vi "cDAQ GET Module Temps.vi"(7 "NI Card Settings":T1, 8 "error in (no error)":errorcluster, 10 "Module Number":i32, 11 "Tasks (In)":refnum<k21>[](array[refnum])) -> (0 "error out":errorcluster, 1 "Raw Data":dbl[](array[numeric]) format="%0.2f", 2 "NI Module Data":string[][](array[string]), 3 "Tasks (Out)":refnum<k21>[](array[refnum]))   [LabVIEW 2019]
uses:
  Trunk/Washer DOE/Type Definitions/DOE Dryer NI Card Settings.ctl
  <vilib>/DAQmx/read.llb/DAQmx Read (Analog 1D DBL NChan 1Samp).vi
  <vilib>/DAQmx/miscellaneous.llb/DAQmx Fill In Error Info.vi
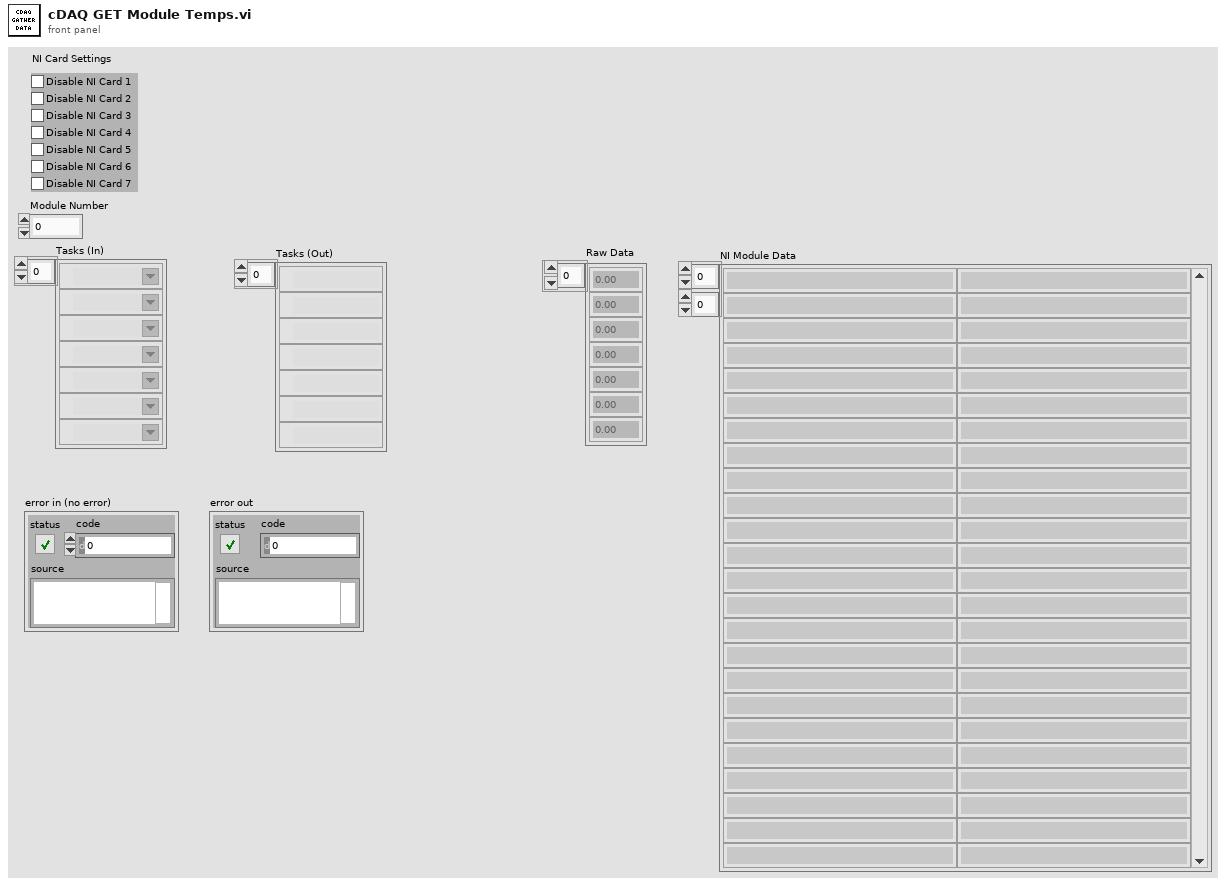
[diagram p1: front panel]
types:
  T1 = typedef "DOE Dryer NI Card Settings.ctl" = cluster{"Disable NI Card 1":bool, "Disable NI Card 2":bool, "Disable NI Card 3":bool, "Disable NI Card 4":bool, "Disable NI Card 5":bool, "Disable NI Card 6":bool, "Disable NI Card 7":bool}
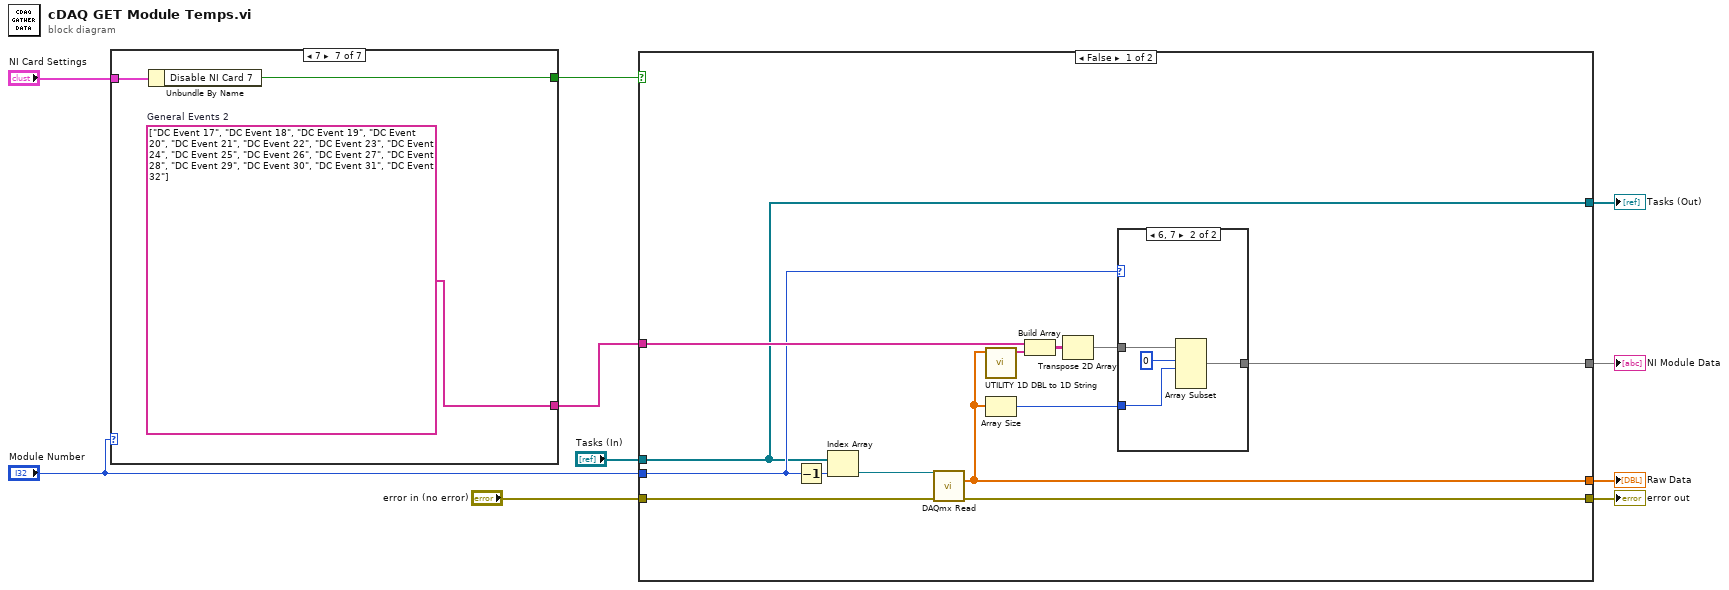
[diagram p0: block diagram]
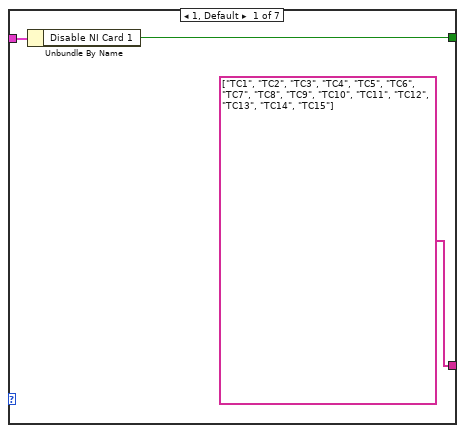
[diagram p2: hidden frame]
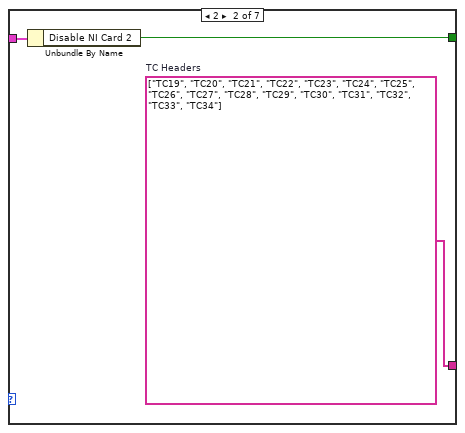
[diagram p3: hidden frame]
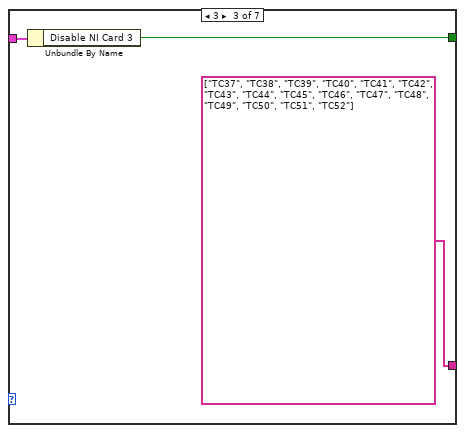
[diagram p4: hidden frame]
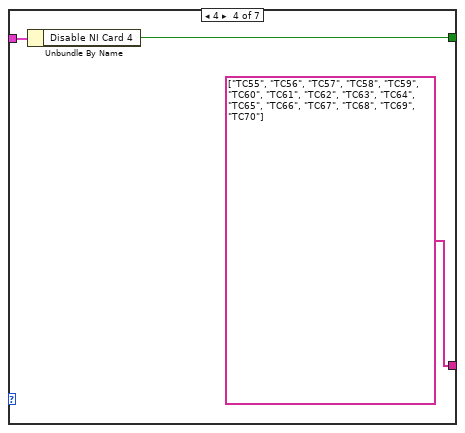
[diagram p5: hidden frame]
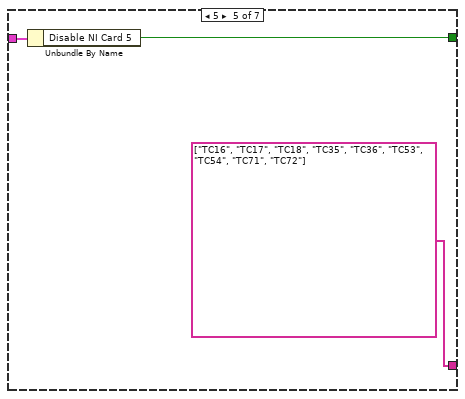
[diagram p6: hidden frame]
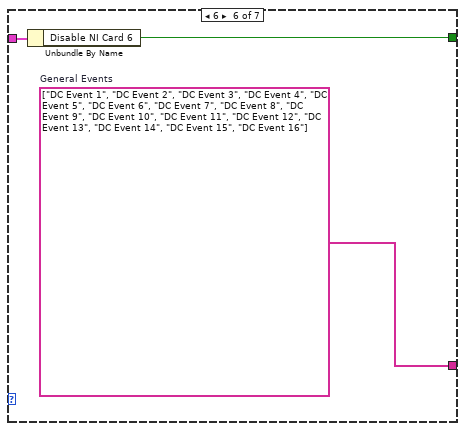
[diagram p7: hidden frame]
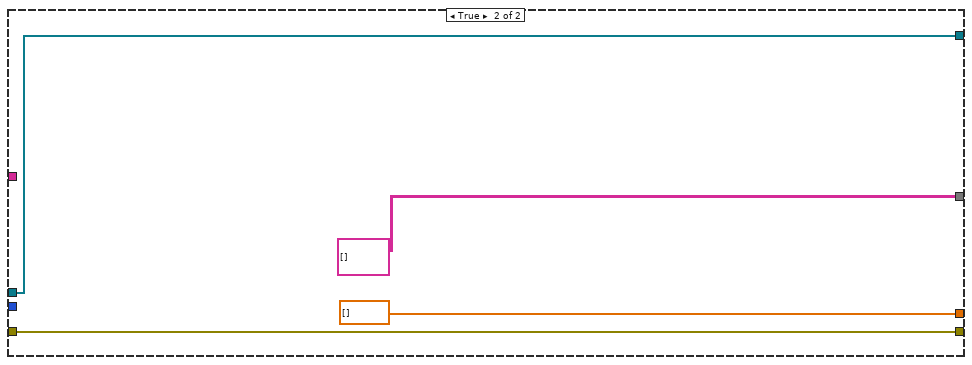
[diagram p9: hidden frame]
diagram:
  n1 = case shown="7" "Module Number" {
    tunnel: "NI Card Settings" -> [w13 w16 w19 w22 w25 w28 w31]
    tunnel: [w12 w15 w18 w21 w24 w27 w30] -> w4
    tunnel: [string[] ["TC1", "TC2", "TC3", "TC4", "TC5", "TC6", "TC7", "TC8", "TC9", "TC10", "TC11", "TC12", "TC13", "TC14", "TC15"] w14 string[] ["TC37", "TC38", "TC39", "TC40", "TC41", "TC42", "TC43", "TC44", "TC45", "TC46", "TC47", "TC48", "TC49", "TC50", "TC51", "TC52"] string[] ["TC55", "TC56", "TC57", "TC58", "TC59", "TC60", "TC61", "TC62", "TC63", "TC64", "TC65", "TC66", "TC67", "TC68", "TC69", "TC70"] string[] ["TC16", "TC17", "TC18", "TC35", "TC36", "TC53", "TC54", "TC71", "TC72"] w26 w29] -> w2
    frame 1, Default {
      n2 = Unbundle By Name(w13) -> ("Disable NI Card 1"=w12:bool)
    }
    frame 2 {
      w14 = string[] ["TC19", "TC20", "TC21", "TC22", "TC23", "TC24", "TC25", "TC26", "TC27", "TC28", "TC29", "TC30", "TC31", "TC32", "TC33", "TC34"]  # TC Headers
      n3 = Unbundle By Name(w16) -> ("Disable NI Card 2"=w15:bool)
    }
    frame 3 {
      n4 = Unbundle By Name(w19) -> ("Disable NI Card 3"=w18:bool)
    }
    frame 4 {
      n5 = Unbundle By Name(w22) -> ("Disable NI Card 4"=w21:bool)
    }
    frame 5 {
      n6 = Unbundle By Name(w25) -> ("Disable NI Card 5"=w24:bool)
    }
    frame 6 {
      w26 = string[] ["DC Event 1", "DC Event 2", "DC Event 3", "DC Event 4", "DC Event 5", "DC Event 6", "DC Event 7", "DC Event 8", "DC Event 9", "DC Event 10", "DC Event 11", "DC Event 12", "DC Event 13", "DC Event 14", "DC Event 15", "DC Event 16"]  # General Events
      n7 = Unbundle By Name(w28) -> ("Disable NI Card 6"=w27:bool)
    }
    frame 7 {
      w29 = string[] ["DC Event 17", "DC Event 18", "DC Event 19", "DC Event 20", "DC Event 21", "DC Event 22", "DC Event 23", "DC Event 24", "DC Event 25", "DC Event 26", "DC Event 27", "DC Event 28", "DC Event 29", "DC Event 30", "DC Event 31", "DC Event 32"]  # General Events 2
      n8 = Unbundle By Name(w31) -> ("Disable NI Card 7"=w30:bool)
    }
  }
  n9 = case shown="False" w4 {
    tunnel: "Tasks (In)" -> [w33 w51]
    tunnel: "error in (no error)" -> [w44 w52]
    tunnel: "Module Number" -> [w34 _]
    tunnel: [w38 dbl[] [] ("data")] -> w8
    tunnel: [w42 w52] -> w7
    tunnel: [w33 w51] -> w3
    tunnel: w2 -> [w40 _]
    tunnel: [w36 string[][] []] -> w1
    frame False {
      n10 = Decrement(x=w34) -> (x-1=w43:i32)
      n11 = Index Array(array=w33, index=w43) -> (element=w32:refnum<k21>)
      n12 = call-poly <vilib>:"DAQmx Read.vi"("task/channels in"=w32, "error in"=w44) -> ("data"=w38:dbl[], "error out"=w42:errorcluster)  [unwired: 11 in, 1 out]
      n13 = call "UTILITY 1D DBL to 1D String.vi"("1D DBL"=w38) -> ("1D String"=w39:string[])  [unwired: 10 in]
      n14 = Array Size(array=w38) -> (size(s)=w35:i32)
      n15 = Build Array(w40, w39) -> (w41:string[][])
      n16 = Transpose 2D Array(2D array=w41) -> (transposed array=w37:string[][])
      n17 = case shown="6, 7" w34 {
        tunnel: w37 -> [w45 w48]
        tunnel: [w45 w47] -> w36
        tunnel: w35 -> [_ w46]
        frame Default {
        }
        frame 6, 7 {
          n18 = Array Subset(array=w48, index (row)=0 ("index"), length (row)=w46) -> (w47:string[][])  [unwired: 2 in]
        }
      }
    }
    frame True {
    }
  }
  "error out" <- w7
  "Raw Data" <- w8
  "Tasks (Out)" <- w3
  "NI Module Data" <- w1
